vi "niTuner Get Temperature.vi"(8 "error in":errorcluster, 9 "correction units":T1(ring)=enum."dBm", 10 "temperature scale":enum16{"Celsius", "Fahrenheit"}(ring), 11 "taskID in":i32=1 format="%.0x") -> (0 "error out":errorcluster {"code" format="%.0x"}, 1 "temperature":dbl format="%.2f", 2 "correction factor":dbl format="%.2p", 3 "taskID out":i32=1 format="%.0x")   [LabVIEW 2011]
doc: "This VI returns the PXI-5600 downconverter temperature in selected units and a factor for correcting the temperature response of the PXI-5600 downconverter."
uses:
  nipxi5600u.dll
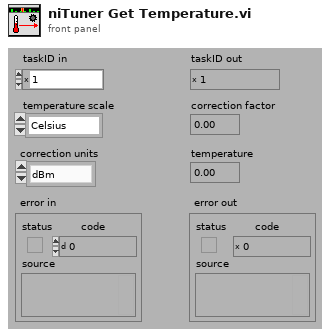
[diagram p1: front panel]
types:
  T1 = enum16{"V", "V^2", "W", "dBm", "dBW", "dBV", "dBmV", "dBuV"}
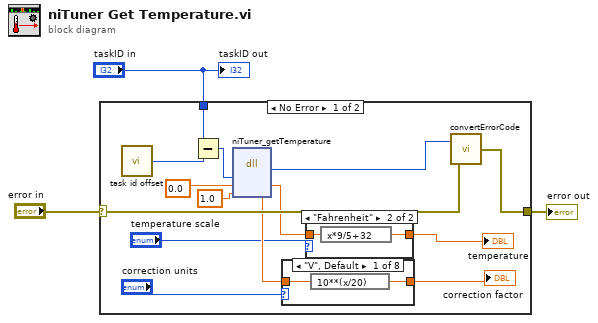
[diagram p0: block diagram]
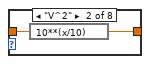
[diagram p3: hidden frame]
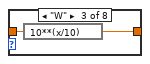
[diagram p4: hidden frame]
diagram:
  n1 = case shown="No Error" "error in" {
    selector: "error in" -> [w16 w32]
    tunnel: [w15 w32] -> w2
    tunnel: "taskID in" -> [w14 _]
    frame No Error {
      n2 = call <instrlib>:"task id offset.vi"() -> ("taskID offset"=w13:i32)
      n3 = Subtract(x=w14, y=w13) -> (x-y=w12:i32)
      n4 = dll-call lib="nipxi5600u.dll" fn="niTuner_getTemperature"("taskID"=w12, "temperature"=0.0 ("taskID"), "tempCorrectionFactor"=1.0) -> (w17:i32, "temperature"=w4:dbl, "tempCorrectionFactor"=w9:dbl)  [unwired: 4 in, 2 out]
      n5 = case shown="\"V\", Default" "correction units" {
        tunnel: w9 -> [w22 w24 w26 w27 w28 w29 w30 w31]
        tunnel: [w21 w23 w25 w27 w28 w29 w30 w31] -> w7
        frame "V", Default {
          n6 = expression code="10**(x/20)"(w22) -> (w21:dbl)
        }
        frame "V^2" {
          n7 = expression code="10**(x/10)"(w24) -> (w23:dbl)
        }
        frame "W" {
          n8 = expression code="10**(x/10)"(w26) -> (w25:dbl)
        }
        frame "dBm" {
        }
        frame "dBW" {
        }
        frame "dBV" {
        }
        frame "dBmV" {
        }
        frame "dBuV" {
        }
      }
      "correction factor" <- w7
      n9 = case shown="\"Fahrenheit\"" "temperature scale" {
        tunnel: w4 -> [w18 w20]
        tunnel: [w18 w19] -> w5
        frame "Celsius", Default {
        }
        frame "Fahrenheit" {
          n10 = expression code="x*9/5+32"(w20) -> (w19:dbl)
        }
      }
      "temperature" <- w5
      n11 = call <instrlib>:"convertErrorCode.vi"("error in"=w16, "error code"=w17) -> ("error out"=w15:errorcluster)
    }
    frame Error {
    }
  }
  "error out" <- w2
  "taskID out" <- "taskID in"
